vi "RSZVB Set TRM User Measurement Path Extension State.vi"(7 "User Measurement Path Extension (Off)":bool, 8 "error in (no error)":errorcluster {"code" format="%.0x"}, 9 "Path (1)":i32=1, 10 "Channel (1)":i32=1, 11 "VISA resource name":refnum<visa-resource-name>) -> (0 "error out":errorcluster {"code" format="%.0x"}, 3 "VISA resource name out":refnum<visa-resource-name>)   [LabVIEW 2011]
doc: "This VI enables/disables the user measurement path extension for RF signal path <Path>.\n\nRemote-control command(s):\n[SENSe<Ch>:]TEUNit:UMEas<Path>[:STATe]"
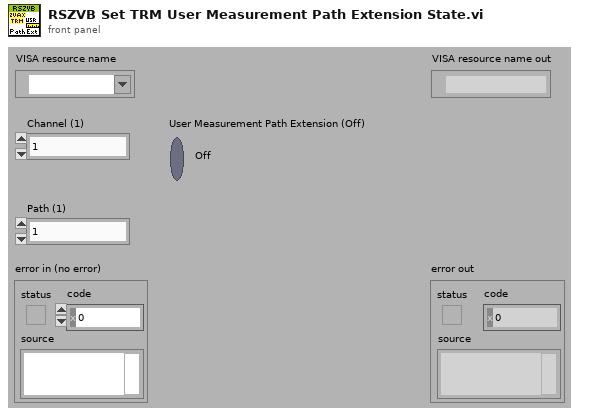
[diagram p1: front panel]
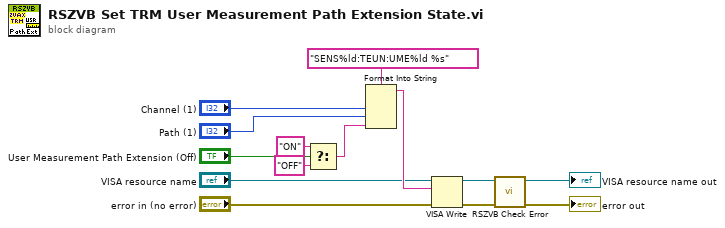
[diagram p0: block diagram]
diagram:
  n1 = Select(t="ON", s="User Measurement Path Extension (Off)", f="OFF") -> (s? t:f=w10:string)
  n2 = Format Into String(format string="SENS%ld:TEUN:UME%ld %s", "Channel (1)", "Path (1)", w10) -> (resulting string=w9:string)  [unwired: 2 in, 1 out]
  n3 = VISA Write(VISA resource name="VISA resource name", write buffer=w9, error in (no error)="error in (no error)") -> (VISA resource name out=w13:refnum<visa-resource-name>, error out=w14:errorcluster)  [unwired: 1 out]
  n4 = call "RSZVB Check Error.vi"("error in (no error)"=w14, "VISA session"=w13) -> ("error out"=→"error out":errorcluster, "dup VISA session"=→"VISA resource name out":refnum<visa-resource-name>)  [unwired: 8 in]
